vi "Pre-Build VI - Run Unit Tests.vi"(8 "error in (no error)":errorcluster) -> (0 "error out":errorcluster, 1 "VIs without test coverage":string[](array[string]), 2 "error type":enum16{"fatal", "non-fatal", "warning"}(ring), 4 "VIs not loadable":string[](array[string]))   [LabVIEW 2009]
uses:
  <userlib>/_OpenG.lib/array/array.llb/Conditional Auto-Indexing Tunnel (String)__ogtk.vi
  <userlib>/_OpenG.lib/array/array.llb/Filter 1D Array (String)__ogtk.vi
panel:
  in  "type specifier VI Refnum (for type only)":refnum<vi>
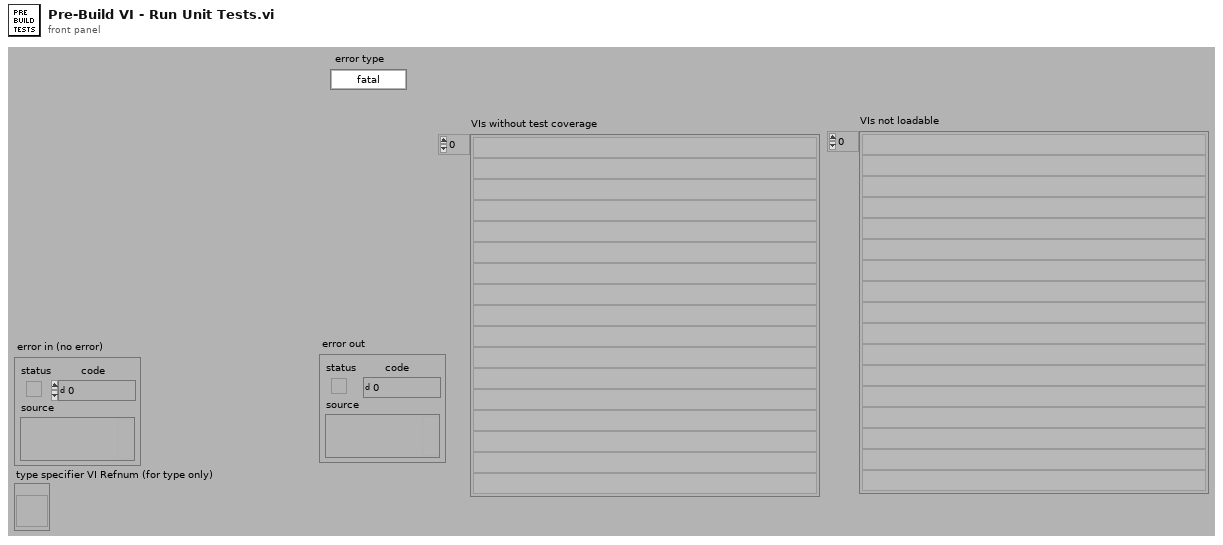
[diagram p1: front panel]
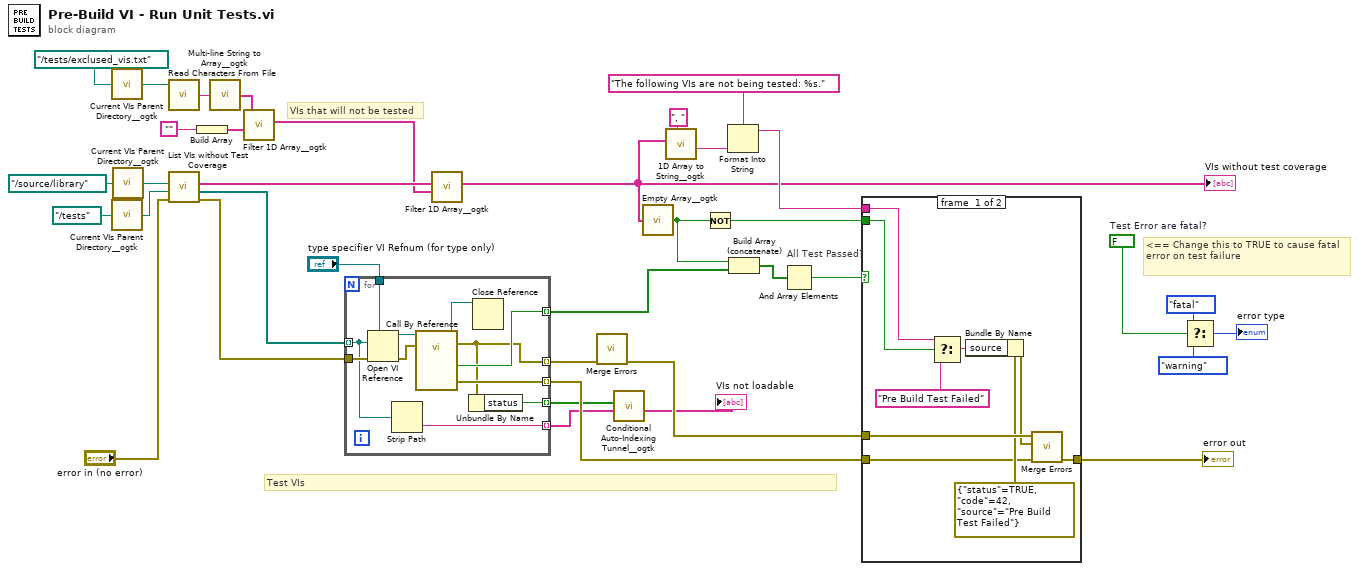
[diagram p0: block diagram]
diagram:
  w24 = FALSE  # Test Error are fatal?
  # "VIs that will not be tested"
  # "<== Change this to TRUE to cause fatal error on test failure"
  # "All Test Passed?"
  # "Test VIs"
  n1 = call <userlib>:"Current VIs Parent Directory__ogtk.vi"("Relative path (.)"=path "../tests/exclused_vis.txt") -> ("Parent Directory (+ Relative)"=w12:path)  [unwired: 4 in]
  n2 = call <userlib>:"Current VIs Parent Directory__ogtk.vi"("Relative path (.)"=path "../tests") -> ("Parent Directory (+ Relative)"=w18:path)  [unwired: 4 in]
  n3 = call <userlib>:"Current VIs Parent Directory__ogtk.vi"("Relative path (.)"=path "../source/library") -> ("Parent Directory (+ Relative)"=w28:path)  [unwired: 4 in]
  n4 = call <vilib>:"Read Characters From File.vi"("file path (dialog if empty)"=w12) -> ("character string"=w11:string)  [unwired: 5 in, 3 out]
  n5 = call "List VIs without Test Coverage.vi"("error in (no error)"="error in (no error)", "Tests Root"=w18, "Source Root"=w28) -> ("error out"=w6:errorcluster, "Test VIs"=w17:path[], "VIs without test coverage"=w35:string[])  [unwired: 6 in]
  n6 = Build Array("") -> (w8:string[])
  n7 = call <userlib>:"Multi-line String to Array__ogtk.vi"("string"=w11) -> ("lines"=w10:string[])
  n8 = call-poly <userlib>:"Filter 1D Array__ogtk.vi"("Items to Filter"=w8, "String Array"=w10) -> ("Filtered String Array"=w7:string[])  [unwired: 5 in]
  n9 = for {
    tunnel: w17 -> [w39] mode=indexing
    tunnel: "type specifier VI Refnum (for type only)" -> [w48]
    tunnel: [w45] -> w15 mode=indexing
    tunnel: [w43] -> w14 mode=indexing
    tunnel: w6 -> [w42]
    tunnel: [w41] -> w4 mode=indexing
    tunnel: [w40] -> w3 mode=indexing
    tunnel: [w38] -> w2 mode=indexing
    n10 = Open VI Reference(type specifier VI Refnum (for type only)=w48, vi path=w39, error in (no error)=w42) -> (vi reference=w47:refnum<vi>, error out=w46:errorcluster)  [unwired: 3 in]
    n11 = Strip Path(path=w39) -> (name=w38:string)  [unwired: 1 out]
    n12 = call-by-ref "?"(reference=w47, error in=w46) -> (reference out=w44:refnum<vi>, error out=w41:errorcluster, 0:"error out"=w43:errorcluster, "pass"=w45:bool)  [unwired: 10 in]
    n13 = Unbundle By Name(w41) -> ("status"=w40:bool)
    n14 = Close Reference(reference=w44) -> ()  [unwired: 1 in, 1 out]
  }
  n15 = call-poly <userlib>:"Filter 1D Array__ogtk.vi"("Items to Filter"=w7, "String Array"=w35) -> ("Filtered String Array"=w20:string[])  [unwired: 5 in]
  "VIs without test coverage" <- w20
  n16 = call <vilib>:"Merge Errors.vi"("error array in"=w4) -> ("error out"=w5:errorcluster)  [unwired: 6 in]
  n17 = call-poly <userlib>:"Conditional Auto-Indexing Tunnel__ogtk.vi"("Array in"=w2, "Elements to keep"=w3) -> ("Filtered Array out"=→"VIs not loadable":string[])  [unwired: 5 in]
  n18 = call <userlib>:"Empty Array__ogtk.vi"("Array"=w20) -> ("Empty Array?"=w30:bool)  [unwired: 8 in]
  n19 = call <userlib>:"1D Array to String__ogtk.vi"("delimiter (Tab)"=", ", "Array of Strings"=w20) -> ("delimited string"=w33:string)  [unwired: 9 in]
  n20 = Not(x=w30) -> (.not. x?=w29:bool)
  n21 = Format Into String(format string="The following VIs are not being tested: %s.", w33) -> (resulting string=w31:string)  [unwired: 2 in, 1 out]
  n22 = Build Array (concatenate)(w30, w15) -> (w37:bool[])
  n23 = And Array Elements(Boolean array=w37) -> (logical AND=w36:bool)
  n24 = case shown="False" w36 {
    tunnel: w5 -> [w57 w58]
    tunnel: [w56 w58] -> w26
    tunnel: w29 -> [w55 _]
    tunnel: w31 -> [w54 _]
    tunnel: w14 -> [w49 _]
    frame #0 {
      n25 = Select(t=w54, s=w55, f="Pre Build Test Failed" ("source")) -> (s? t:f=w52:string)
      n26 = Bundle By Name(cluster=errorcluster {"status"=TRUE, "code"=42, "source"="Pre Build Test Failed"} ("error out"), "source"=w52) -> (w51:errorcluster)
      n27 = call <vilib>:"Merge Errors.vi"("error array in"=w49, "error in 2 (no error)"=w51, "error in 1 (no error)"=w57) -> ("error out"=w56:errorcluster)  [unwired: 4 in]
    }
    frame #1 {
    }
  }
  "error out" <- w26
  n28 = Select(t=enum16{"fatal", "non-fatal", "warning"}."fatal" ("error type"), s=w24, f=enum16{"fatal", "non-fatal", "warning"}."warning" ("error type")) -> (s? t:f=→"error type":enum16{"fatal", "non-fatal", "warning"})
